vi "Create FPGA Direct IO.vi"(8 "error in (no error)":errorcluster, 11 "FPGA Interface":refnum<k20>) -> (0 "error out":errorcluster, 3 "FPGA direct IO out":refnum<class "NI_Robotics_Starter Kit Direct IO_FPGA.lvclass">)   [LabVIEW 2017, in "NI_Robotics_Starter Kit Direct IO_FPGA.lvclass"]
uses:
  <vilib>/robotics/Starter Kit/FPGA Direct IO/NI_Robotics_Starter Kit Direct IO_FPGA.lvclass
  c:/Program Files (x86)/National Instruments/LabVIEW 2017/vi.lib/robotics/Starter Kit/Base Device/NI_Robotics_Starter Kit Base Device.lvclass
  <vilib>/robotics/Starter Kit/FPGA Direct IO/Direct IO FPGA Ref.ctl
  <vilib>/robotics/Starter Kit/FPGA Direct IO/NI_Robotics_Starter Kit Direct IO_FPGA.lvclass/NI_Robotics_Starter Kit Direct IO_FPGA.ctl
  <vilib>/robotics/Starter Kit/Base Device/NI_Robotics_Starter Kit Base Device.lvclass/NI_Robotics_Starter Kit Base Device.ctl
  <vilib>/robotics/Starter Kit/Base Device/NI_Robotics_Starter Kit Base Device.lvclass
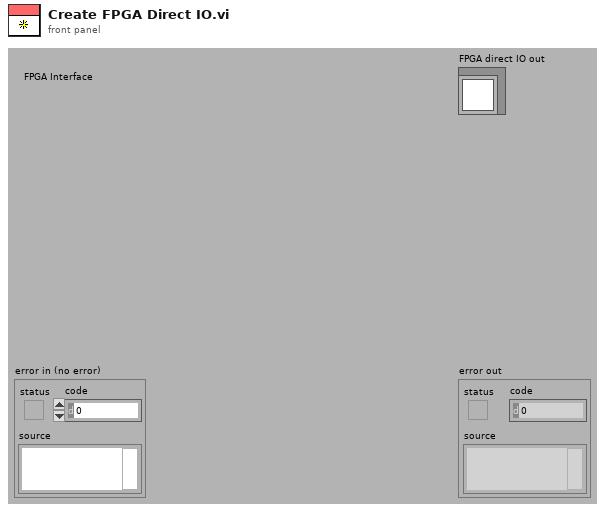
[diagram p1: front panel]
types:
  T1 = typedef "NI_Robotics_Starter Kit Direct IO_FPGA.lvclass/Direct IO FPGA Ref.ctl" = refnum<k20>
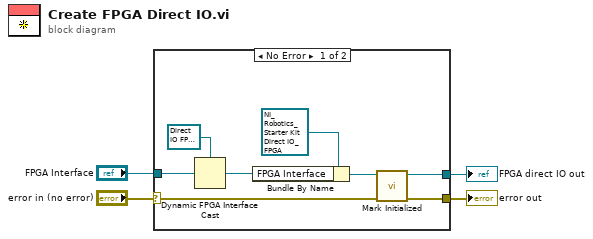
[diagram p0: block diagram]
diagram:
  n1 = case shown="No Error" "error in (no error)" {
    selector: "error in (no error)" -> [w9 w13]
    tunnel: [w8 w13] -> w3
    tunnel: [w10 _] -> w2
    tunnel: "FPGA Interface" -> [w7 _]
    frame No Error {
      n2 = Dynamic FPGA Interface Cast(Session In=T1 refnum ("FPGA Interface"), Type=w7) -> (Session Out=w5:T1)
      n3 = Bundle By Name(cluster=refnum<class "NI_Robotics_Starter Kit Direct IO_FPGA.lvclass"> refnum ("FPGA direct IO out"), "FPGA Interface"=w5) -> (w11:refnum<class "NI_Robotics_Starter Kit Direct IO_FPGA.lvclass">)
      n4 = call <vilib>:"Mark Initialized.vi"("error in (no error)"=w9, "device in"=w11) -> ("error out"=w8:errorcluster, "device out"=w10:refnum<class "NI_Robotics_Starter Kit Direct IO_FPGA.lvclass">)  [unwired: 8 in]
    }
    frame Error {
    }
  }
  "error out" <- w3
  "FPGA direct IO out" <- w2
